vi "Telnet Buffered Read.vi"(7 "unfiltered buffer in":string, 8 "error in (no error)":errorcluster, 9 "read info":T1={"bytes to read"=60, "timeout ms"=100, "read mode"=enum."normal", "line separator"="login: "}, 10 "buffer in":string, 11 "connection ID":refnum<k5>) -> (0 "error out":errorcluster, 1 "data":string, 2 "buffer out":string, 3 "connection ID out":refnum<k5>, 4 "unfiltered buffer out":string)   [LabVIEW 2014]
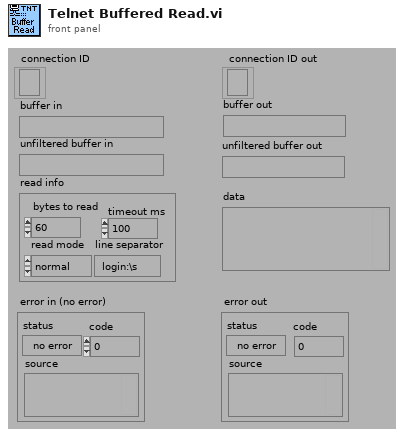
[diagram p1: front panel]
types:
  T1 = cluster{"bytes to read":i32, "timeout ms":i32, "read mode":enum16{"normal", "line", "buffered"}, "line separator":string}
  T2 = enum16{"Standard", "Buffered", "CRLF", "Immediate"}
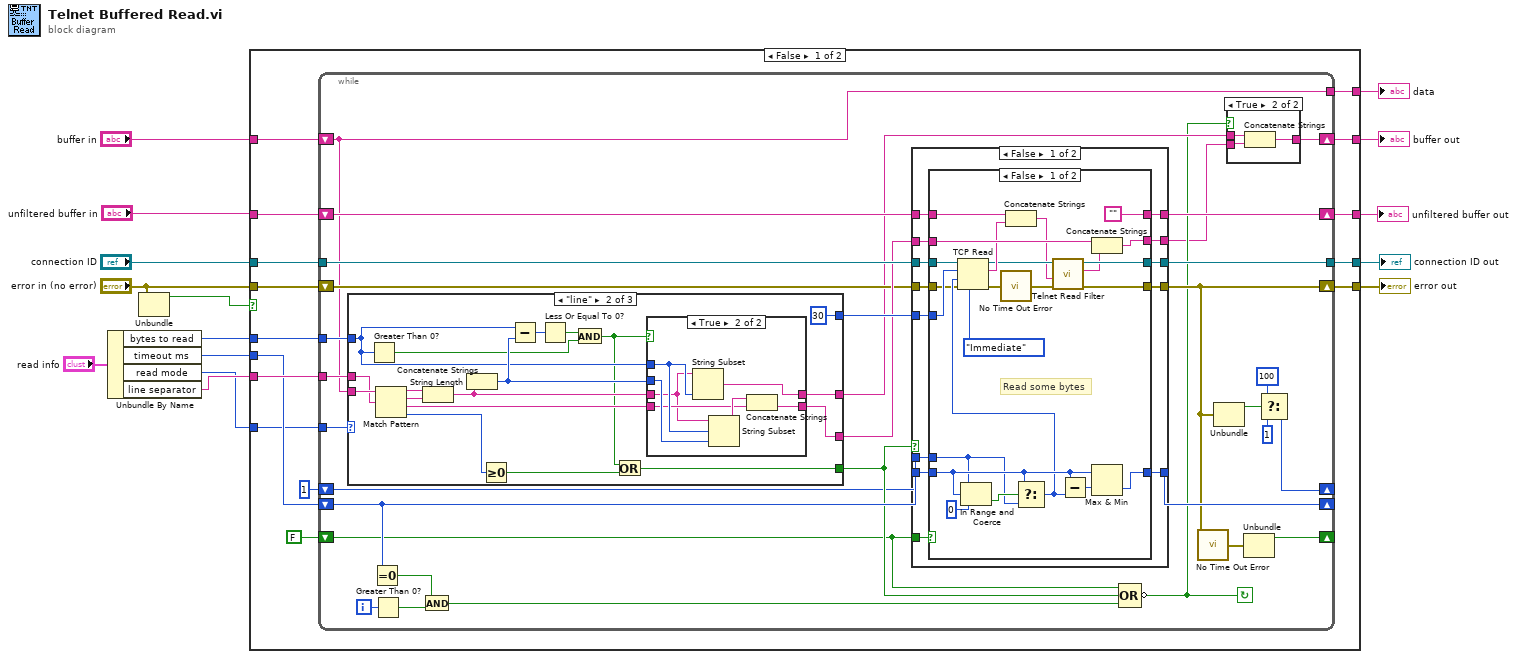
[diagram p0: block diagram]
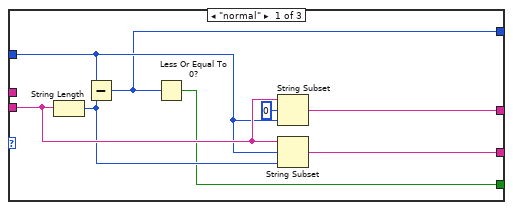
[diagram p3: hidden frame]
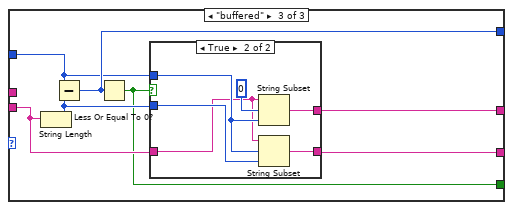
[diagram p5: hidden frame]
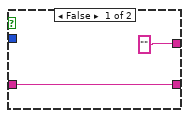
[diagram p6: hidden frame]
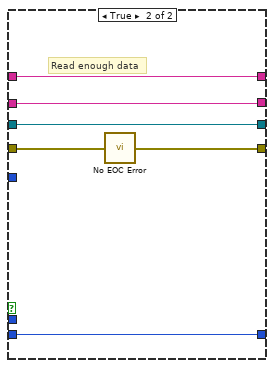
[diagram p8: hidden frame]
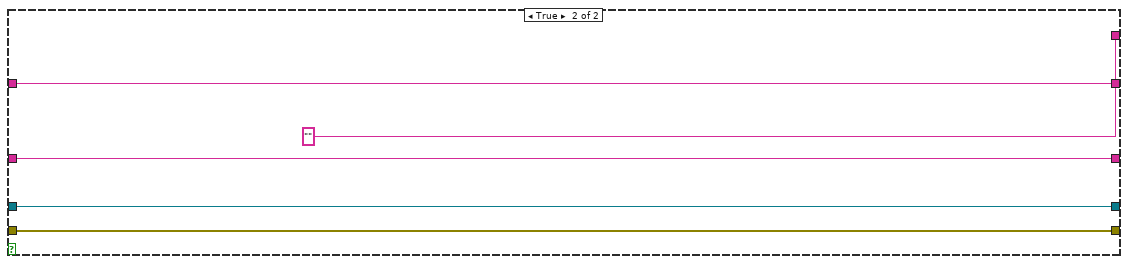
[diagram p9: hidden frame]
diagram:
  n1 = Unbundle By Name("read info") -> ("bytes to read"=w14:i32, "timeout ms"=w13:i32, "read mode"=w10:enum16{"normal", "line", "buffered"}, "line separator"=w12:string)
  n2 = Unbundle("error in (no error)") -> ("status"=w9:bool)  [unwired: 2 out]
  n3 = case shown="False" w9 {
    tunnel: "buffer in" -> [w30 w165]
    tunnel: w14 -> [w19 _]
    tunnel: w13 -> [w27 _]
    tunnel: "connection ID" -> [w28 w164]
    tunnel: w12 -> [w29 _]
    tunnel: "error in (no error)" -> [w18 w167]
    tunnel: [w26 w164] -> w2
    tunnel: [w17 w167] -> w4
    tunnel: [w25 w165] -> w3
    tunnel: "unfiltered buffer in" -> [w23 w166]
    tunnel: [w22 w166] -> w11
    tunnel: w10 -> [w20 _]
    tunnel: [w16 "" ("substring")] -> w1
    frame False {
      n4 = while {
        tunnel: [w31] -> w16
        shift-right: [w32] -> w25
        shift-left: w30 -> [w31]
        tunnel: w29 -> [w61]
        tunnel: w28 -> [w60]
        shift-right: [w59] -> _
        shift-left: w27 -> [w57]
        tunnel: [w58] -> w26
        shift-right: [w47] -> _
        shift-left: FALSE ("status") -> [w51]
        shift-right: [w49] -> w22
        shift-left: w23 -> [w50]
        shift-right: [w42] -> _
        shift-left: 1 ("bytes to read") -> [w46]
        tunnel: w20 -> [w40]
        tunnel: w19 -> [w39]
        shift-right: [w36] -> w17
        shift-left: w18 -> [w37]
        i -> [w56]
        stop <- w34 continue-if-true
        n5 = case shown="\"line\"" w40 {
          tunnel: [w66 30 ("bytes to read") w102] -> w41
          tunnel: [w72 w80 w106] -> w35
          tunnel: [w69 w83 w103] -> w52
          tunnel: w31 -> [w73 w89 w107]
          tunnel: [w70 w79 w104] -> w38
          tunnel: w61 -> [_ w87 _]
          tunnel: w39 -> [w67 w77 w101]
          frame "normal" {
            n6 = String Length(string=w73) -> (length=w71:i32)
            n7 = Subtract(x=w67, y=w71) -> (x-y=w66:i32)
            n8 = Less Or Equal To 0?(x=w66) -> (x <= 0?=w69:bool)
            n9 = String Subset(string=w73, offset (0)=0 ("length"), length (rest)=w67) -> (substring=w72:string)
            n10 = String Subset(string=w73, offset (0)=w67, length (rest)=w71) -> (substring=w70:string)
          }
          frame "line" {
            n11 = Greater Than 0?(x=w77) -> (x > 0?=w74:bool)
            n12 = Match Pattern(string=w89, regular expression=w87) -> (before substring=w88:string, match substring=w90:string, after substring=w81:string, offset past match=w86:i32)  [unwired: 1 in]
            n13 = Concatenate Strings(w88, w90) -> (w82:string)
            n14 = String Length(string=w82) -> (length=w78:i32)
            n15 = Greater Or Equal To 0?(x=w86) -> (x >= 0?=w84:bool)
            n16 = Subtract(x=w77, y=w78) -> (x-y=w85:i32)
            n17 = Less Or Equal To 0?(x=w85) -> (x <= 0?=w75:bool)
            n18 = And(x=w75, y=w74) -> (x .and. y?=w76:bool)
            n19 = Or(x=w76, y=w84) -> (x .or. y?=w83:bool)
            n20 = case shown="True" w76 {
              tunnel: w82 -> [w93 w95]
              tunnel: w81 -> [w92 w97]
              tunnel: [w93 w94] -> w80
              tunnel: [w92 w96] -> w79
              tunnel: w77 -> [_ w100]
              tunnel: w78 -> [_ w99]
              frame False {
              }
              frame True {
                n21 = String Subset(string=w95, length (rest)=w100) -> (substring=w94:string)  [unwired: 1 in]
                n22 = String Subset(string=w95, offset (0)=w100, length (rest)=w99) -> (substring=w98:string)
                n23 = Concatenate Strings(w98, w97) -> (w96:string)
              }
            }
          }
          frame "buffered" {
            n24 = String Length(string=w107) -> (length=w105:i32)
            n25 = Subtract(x=w101, y=w105) -> (x-y=w102:i32)
            n26 = Less Or Equal To 0?(x=w102) -> (x <= 0?=w103:bool)
            n27 = case shown="True" w103 {
              tunnel: [w109 w115] -> w104
              tunnel: w105 -> [_ w114]
              tunnel: ["" ("substring") w113] -> w106
              tunnel: w107 -> [w109 w110]
              tunnel: w101 -> [_ w112]
              frame False {
              }
              frame True {
                n28 = String Subset(string=w110, offset (0)=0 ("length"), length (rest)=w112) -> (substring=w113:string)
                n29 = String Subset(string=w110, offset (0)=w112, length (rest)=w114) -> (substring=w115:string)
              }
            }
          }
        }
        n30 = Equal To 0?(x=w57) -> (x = 0?=w55:bool)
        n31 = Greater Than 0?(x=w56) -> (x > 0?=w54:bool)
        n32 = And(x=w55, y=w54) -> (x .and. y?=w53:bool)
        n33 = case shown="False" w52 {
          tunnel: [w126 w157] -> w33
          tunnel: w38 -> [w128 w157]
          tunnel: [w120 w160] -> w36
          tunnel: w60 -> [w127 w161]
          tunnel: w57 -> [w124 w162]
          tunnel: [w123 w162] -> w59
          tunnel: [w125 w161] -> w58
          tunnel: w51 -> [w122 _]
          tunnel: w37 -> [w121 w159]
          tunnel: w50 -> [w119 w158]
          tunnel: [w118 w158] -> w49
          tunnel: w46 -> [w117 _]
          tunnel: w41 -> [w116 _]
          frame False {
            n34 = case shown="False" w122 {
              tunnel: [w151 w155] -> w123
              tunnel: w124 -> [w150 w155]
              tunnel: [w131 w156] -> w125
              tunnel: [w139 w152] -> w126
              tunnel: [w133 w154] -> w120
              tunnel: w127 -> [w147 w156]
              tunnel: w128 -> [w146 w152]
              tunnel: w121 -> [w141 w154]
              tunnel: w119 -> [w145 w153]
              tunnel: ["" w153] -> w118
              tunnel: w117 -> [w144 _]
              tunnel: w116 -> [w143 _]
              frame False {
                # "Read some bytes"
                n35 = In Range and Coerce(upper limit=w144, x=w150, lower limit=0 ("bytes to read")) -> (In Range?=w149:bool)  [unwired: 1 out]
                n36 = Select(t=w150, s=w149, f=w144) -> (s? t:f=w142:i32)
                n37 = TCP Read(connection ID=w147, bytes to read=w143, error in (no error)=w141, 7:T2."Immediate" ("mode (standard)"), 9:w142) -> (connection ID out=w132:refnum<k5>, data out=w138:string, error out=w140:errorcluster)
                n38 = call "No Time Out Error.vi"("error in (no error)"=w140) -> ("error out"=w134:errorcluster)  [unwired: 14 in]
                n39 = Concatenate Strings(w145, w138) -> (w130:string)
                n40 = call "Telnet Read Filter.vi"("error in"=w134, "unfiltered data in"=w130, "Connection in"=w132) -> ("error out"=w133:errorcluster, "Data out"=w129:string, "connection out"=w131:refnum<k5>)  [unwired: 1 in, 1 out]
                n41 = Subtract(x=w150, y=w142) -> (x-y=w135:i32)
                n42 = Concatenate Strings(w146, w129) -> (w139:string)
                n43 = Max & Min(x=w150, y=w135) -> (min(x,y)=w151:i32)  [unwired: 1 out]
              }
              frame True {
                # "Error! (Connection closed, etc.)"
              }
            }
          }
          frame True {
            # "Read enough data"
            n44 = call "No EOC Error.vi"("error in (no error)"=w159) -> ("error out"=w160:errorcluster)  [unwired: 4 in]
          }
        }
        n45 = Compound Arithmetic op=OR(w51, w52, w53) -> (invert w34:bool)
        n46 = call "No Time Out Error.vi"("error in (no error)"=w36) -> ("error out"=w48:errorcluster)  [unwired: 14 in]
        n47 = Unbundle(w36) -> ("status"=w45:bool)  [unwired: 2 out]
        n48 = case shown="True" w34 {
          tunnel: w33 -> [w62 w65]
          tunnel: w35 -> [_ w64]
          tunnel: [w62 w63] -> w32
          frame False {
          }
          frame True {
            n49 = Concatenate Strings(w64, w65) -> (w63:string)
          }
        }
        n50 = Unbundle(w48) -> ("status"=w47:bool)  [unwired: 2 out]
        n51 = Select(t=100 ("bytes to read"), s=w45, f=1 ("bytes to read")) -> (s? t:f=w42:i32)
      }
    }
    frame True {
    }
  }
  "error out" <- w4
  "connection ID out" <- w2
  "buffer out" <- w3
  "data" <- w1
  "unfiltered buffer out" <- w11
